vi "Set Buffer and Get Channel Reading DBL.vi"(6 "Timestamps":timestamp[](array[timestamp]) format="%<%x %.3X>T", 8 "error in":errorcluster, 9 "Readings":dbl[][](array[numeric]), 10 "Channel Ident":string, 11 "BufferLastReads in":refnum<class "BufferLastReads.lvclass">) -> (0 "error out":errorcluster, 2 "Last Read":variant, 3 "BufferLastReads out":refnum<class "BufferLastReads.lvclass">)   [LabVIEW 2024, in "BufferLastReads.lvclass"]
uses:
  BufferLastReads.lvclass
  BufferLastReads.lvclass/BufferLastReads.ctl
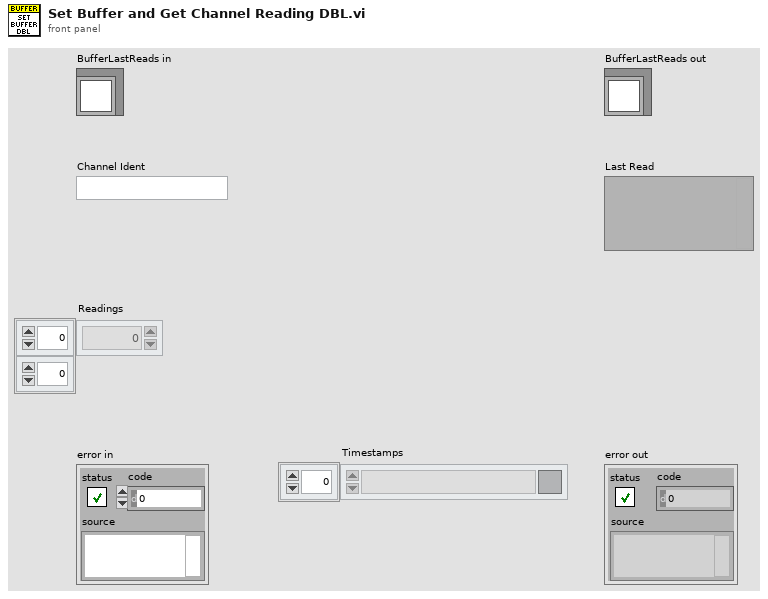
[diagram p1: front panel]
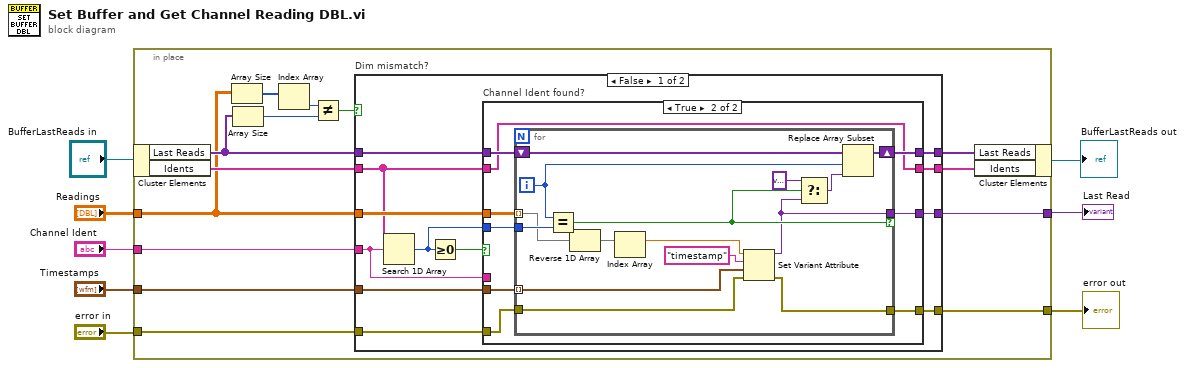
[diagram p0: block diagram]
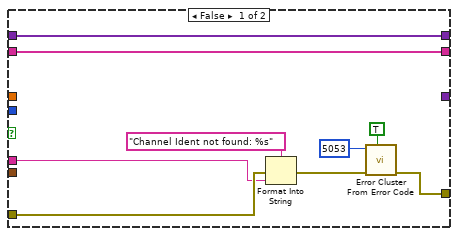
[diagram p2: hidden frame]
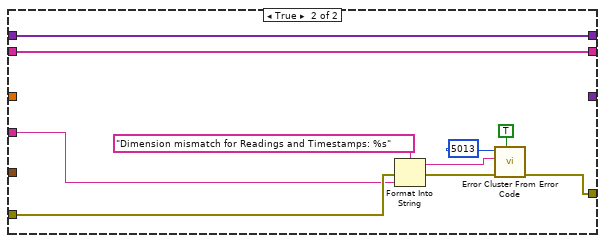
[diagram p3: hidden frame]
diagram:
  n1 = in-place {
    in-place-border: "Readings" -> [w13]
    in-place-border: "Channel Ident" -> [w18]
    in-place-border: "error in" -> [w20]
    in-place-border: [w19] -> w5
    in-place-border: [w17] -> w2
    in-place-border: "Timestamps" -> [w16]
    n2 = in-place-cluster #1("BufferLastReads in") -> ("Last Reads"=w14:variant[], "Idents"=w21:string[])
    n3 = Array Size(array=w13) -> (size(s)=w10:i32[])
    n4 = Array Size(array=w14) -> (size(s)=w11:i32)
    n5 = Index Array(array=w10) -> (element=w9:i32)  [unwired: 1 in]
    n6 = Not Equal?(x=w9, y=w11) -> (x != y?=w12:bool)
    n7 = case "Dim mismatch?" shown="False" w12 {
      tunnel: w13 -> [w34 _]
      tunnel: w14 -> [w33 w68]
      tunnel: [w32 w68] -> w22
      tunnel: w21 -> [w24 w77]
      tunnel: w20 -> [w29 w72]
      tunnel: [w28 w71] -> w19
      tunnel: w18 -> [w27 w70]
      tunnel: [w26 _] -> w17
      tunnel: w16 -> [w25 _]
      tunnel: [w23 w77] -> w15
      frame False {
        n8 = Search 1D Array(1D array=w24, element=w27) -> (index of element=w31:i32)  [unwired: 1 in]
        n9 = Greater Or Equal To 0?(x=w31) -> (x >= 0?=w30:bool)
        n10 = case "Channel Ident found?" shown="True" w30 {
          tunnel: w34 -> [_ w52]
          tunnel: w33 -> [w41 w51]
          tunnel: [w41 w50] -> w32
          tunnel: w31 -> [_ w49]
          tunnel: w29 -> [w39 w48]
          tunnel: [w42 w46] -> w28
          tunnel: w27 -> [w36 _]
          tunnel: w25 -> [_ w47]
          tunnel: [_ w45] -> w26
          tunnel: w24 -> [w35 w44]
          tunnel: [w35 w44] -> w23
          frame False {
            n11 = Format Into String(format string="Channel Ident not found: %s", error in=w39, w36) -> (error out=w38:errorcluster)  [unwired: 1 in, 1 out]
            n12 = call <vilib>:"Error Cluster From Error Code.vi"("show call chain? (False)"=TRUE, "error in (no error)"=w38, "error code (0)"=5053) -> ("error out"=w42:errorcluster)  [unwired: 6 in]
          }
          frame True {
            n13 = for {
              tunnel: [w55] -> w45 if=w67
              tunnel: w52 -> [w60] mode=indexing
              shift-right: [w62] -> w50
              shift-left: w51 -> [w65]
              tunnel: w49 -> [w61]
              tunnel: w48 -> [w58]
              tunnel: w47 -> [w57] mode=indexing
              tunnel: [w56] -> w46
              i -> [w64]
              n14 = Equal?(x=w64, y=w61) -> (x = y?=w67:bool)
              n15 = Reverse 1D Array(array=w60) -> (reversed array=w54:dbl[])
              n16 = Index Array(array=w54) -> (element=w53:dbl)  [unwired: 1 in]
              n17 = Set Variant Attribute(Variant=w53, name="timestamp", value=w57, error in=w58) -> (Variant out=w55:variant, error out=w56:errorcluster)  [unwired: 1 out]
              n18 = Select(t=variant, s=w67, f=w55) -> (s? t:f=w63:variant)
              n19 = Replace Array Subset(array=w65, new element=w63, index=w64) -> (w62:variant[])
            }
          }
        }
      }
      frame True {
        n20 = Format Into String(format string="Dimension mismatch for Readings and Timestamps: %s", error in=w72, w70) -> (resulting string=w69:string, error out=w74:errorcluster)  [unwired: 1 in]
        n21 = call <vilib>:"Error Cluster From Error Code.vi"("show call chain? (False)"=TRUE, "error in (no error)"=w74, "error message (\"\")"=w69, "error code (0)"=5013) -> ("error out"=w71:errorcluster)  [unwired: 5 in]
      }
    }
    n22 = in-place-cluster #1("Last Reads"=w22, "Idents"=w15) -> (→"BufferLastReads out":refnum<class "BufferLastReads.lvclass">)
  }
  "error out" <- w5
  "Last Read" <- w2
